vi "Servo Read system configuration.vi"(8 "error in (no error)":errorcluster, 11 "MAG config file path":path) -> (0 "error out":errorcluster, 1 "User defined path":bool, 3 "IP addresses":string[](array[string]))   [LabVIEW 2024]
doc: "Reads an INI file with magnet configuration data, for example port names and maximum ramp/field constants.\nConsiderable build-in function: searching for SMS serial port"
uses:
  <vilib>/Utility/error.llb/Error Cluster From Error Code.vi
  <vilib>/ErrorRing/Error Ring.xnode
  <vilib>/Utility/config.llb/NI_LVConfig.lvlib
  <userlib>/_OpenG.lib/variantconfig/variantconfig.llb/openg_variant_configuration_file.lvlib
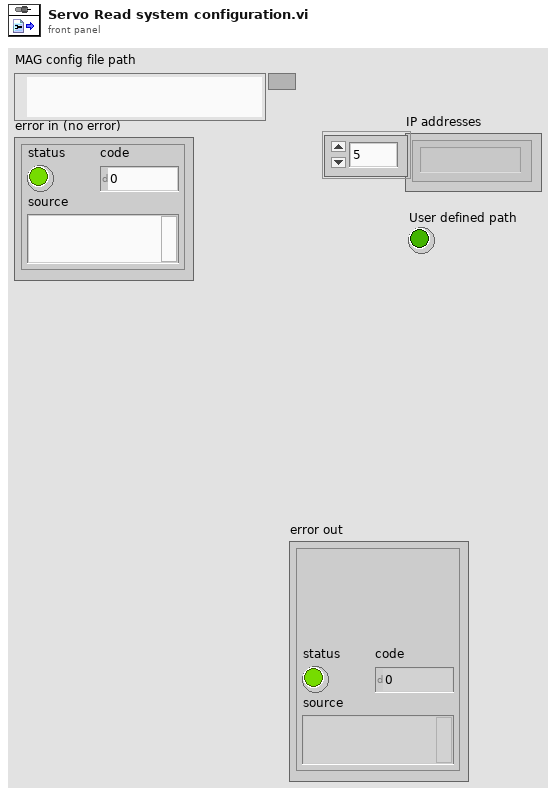
[diagram p1: front panel]
types:
  T1 = typedef "NI_LVConfig.lvlib/Config Data RefNum.ctl" = refnum<k1>
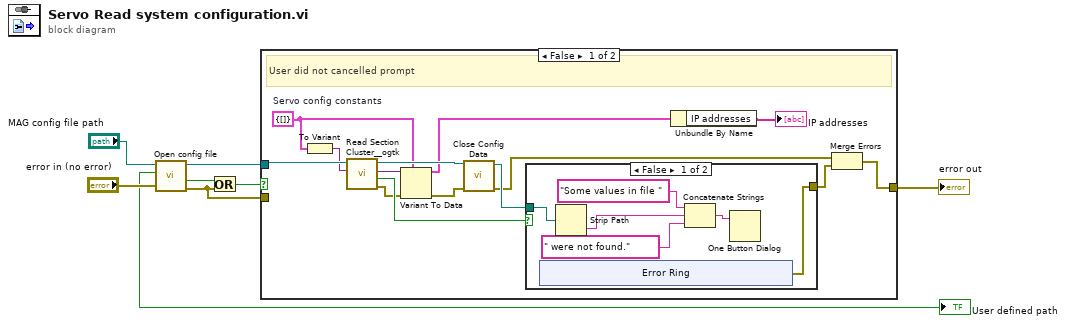
[diagram p0: block diagram]
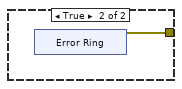
[diagram p2: hidden frame]
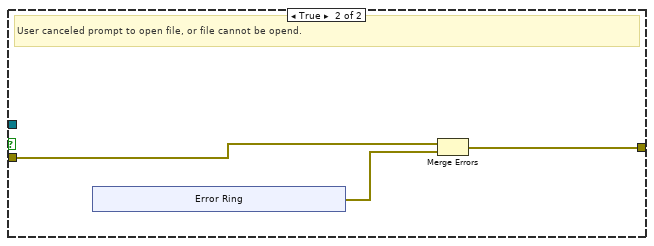
[diagram p3: hidden frame]
diagram:
  n1 = call "Open config file.vi"("error in (no error)"="error in (no error)", "MAG config file path"="MAG config file path") -> ("error out"=w1:errorcluster, "cancelled prompt"=w4:bool, "prompted"=→"User defined path":bool, "Refnum out"=w7:T1)  [unwired: 6 in]
  n2 = Or(x=w4, y=w1) -> (x .or. y?=w2:bool)
  n3 = case shown="False" w2 {
    tunnel: w7 -> [w17 _]
    tunnel: w1 -> [_ w35]
    tunnel: [w12 w36] -> w3
    frame False {
      w15 = cluster{"IP addresses":string[]} {"IP addresses"=[]}  # Servo config constants
      # "User did not cancelled prompt"
      n4 = To Variant(anything=w15) -> (Variant=w16:variant)
      n5 = call <userlib>:"Read Section Cluster__ogtk.vi"("Section Formatted Cluster Type"=w16, "refnum"=w17) -> ("error out"=w19:errorcluster, "all found?"=w21:bool, "Section Formatted Cluster"=w22:variant, "dup refnum"=w20:T1)  [unwired: 5 in, 1 out]
      n6 = Variant To Data(error in=w19, type=w15, Variant=w22) -> (data=w9:cluster{"IP addresses":string[]}, error out=w18:errorcluster)
      n7 = call <vilib>:"Close Config Data.vi"("error in (no error)"=w18, "refnum"=w20) -> ("error out"=w13:errorcluster, "file path"=w14:path)  [unwired: 8 in]
      n8 = case shown="False" w21 {
        tunnel: w14 -> [w26 _]
        tunnel: [w23 w33] -> w11
        frame False {
          n9 = xnode "Error Ring"() -> ("error out"=w23:errorcluster)
          n10 = Strip Path(path=w26) -> (name=w25:string)  [unwired: 1 out]
          n11 = Concatenate Strings("Some values in file " ("message"), w25, " were not found." ("string")) -> (w27:string)
          n12 = One Button Dialog(message=w27) -> ()  [unwired: 1 in, 1 out]
        }
        frame True {
          n13 = xnode "Error Ring"() -> ("error out"=w33:errorcluster)
        }
      }
      n14 = Unbundle By Name(w9) -> ("IP addresses"=→"IP addresses":string[])
      n15 = Merge Errors(w13, w11) -> (w12:errorcluster)
    }
    frame True {
      # "User canceled prompt to open file, or file cannot be opend."
      n16 = xnode "Error Ring"() -> ("error out"=w37:errorcluster)
      n17 = Merge Errors(w35, w37) -> (w36:errorcluster)
    }
  }
  "error out" <- w3
